vi "Serial Config.vi"(8 "error in":errorcluster, 11 "cPAS in":refnum<class "cPAS.lvclass">) -> (0 "error out":errorcluster, 3 "cPAS out":refnum<class "cPAS.lvclass">)   [LabVIEW 2014, in "cPAS.lvclass"]
uses:
  cPAS.lvclass
  Reusable/Serial IO/Serial IO.lvclass
  Devices/TE Cooler/TE Cooler.lvclass
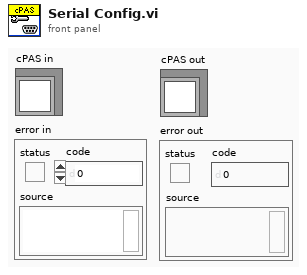
[diagram p1: front panel]
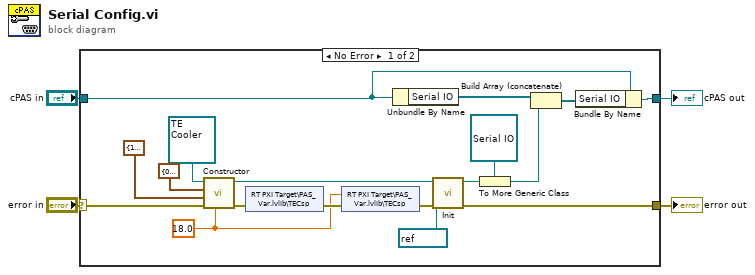
[diagram p0: block diagram]
diagram:
  n1 = case shown="No Error" "error in" {
    selector: "error in" -> [w5 w24]
    tunnel: "cPAS in" -> [w20 w23]
    tunnel: [w21 w23] -> w2
    tunnel: [w9 w24] -> w1
    frame No Error {
      w6 = sgl 18.0 ("TSP")
      n2 = call "Constructor.vi"("TSP"=w6, "error in"=w5, "PID Params"=cluster{"P":sgl, "I":sgl, "D":sgl} {"P"=1.0, "I"=0.75, "D"=0.0}, "Ctl Params"=cluster{"htx":sgl, "clx":sgl} {"htx"=0.0, "clx"=0.75}, "TE Cooler in"=refnum<class "TE Cooler.lvclass"> refnum ("TE Cooler.lvlib:TE Cooler.lvclass")) -> ("error out"=w19:errorcluster, "TE Cooler out"=w16:refnum<class "TE Cooler.lvclass">)  [unwired: 5 in]
      n3 = shared-variable "RT PXI Target\\PAS_Var.lvlib\\TECsp"(error in=w19) -> (error out=w18:errorcluster)  [unwired: 1 out]
      n4 = shared-variable "RT PXI Target\\PAS_Var.lvlib\\TECsp"(w6, error in=w18) -> (error out=w17:errorcluster)
      n5 = Unbundle By Name(w20) -> ("Serial IO"=w11:refnum<class "Configurable Device.lvclass">[])
      n6 = call-dynamic "Init.vi"("error in"=w17, 10:refnum<visa-resource-name> "TEC" ("Port"), "TE Cooler in"=w16) -> ("error out"=w9:errorcluster, "TE Cooler out"=w15:refnum<class "TE Cooler.lvclass">)  [unwired: 7 in]
      n7 = To More Generic Class(target class=refnum<class "Serial IO.lvclass"> refnum ("Serial IO.lvclass"), reference=w15) -> (generic class reference=w12:refnum<class "Serial IO.lvclass">)
      n8 = Build Array (concatenate)(w11, w12) -> (w10:refnum<class>[])
      n9 = Bundle By Name(cluster=w20, "Serial IO"=w10) -> (w21:refnum<class "cPAS.lvclass">)
    }
    frame Error {
    }
  }
  "error out" <- w1
  "cPAS out" <- w2
